vi "Advanced Cut - Auto Reverse Cut.vi"(8 "error in (no error)":errorcluster, 11 "Auto Cut (Reverse)":T1={"End Time (s)"=0.0, "# Epochs"=10, "Epoch Duration (s)"=90.0} {"Epoch Duration (s)" min=0.0 step=1.0; "End Time (s)" min=0.0 step=1.0}) -> (0 "error out":errorcluster, 3 "Snippets":dbl[][](array[numeric]))   [LabVIEW 2016]
uses:
  Type Definitions/Advanced Cut - Reverse Auto Cut.ctl
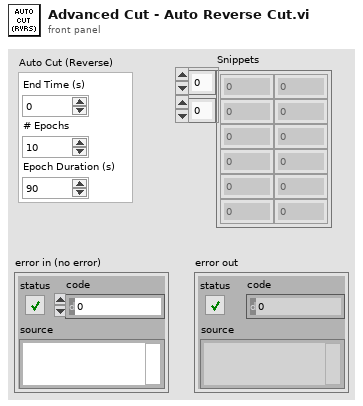
[diagram p1: front panel]
types:
  T1 = typedef "Advanced Cut - Reverse Auto Cut.ctl" = cluster{"End Time (s)":dbl, "# Epochs":u32, "Epoch Duration (s)":dbl}
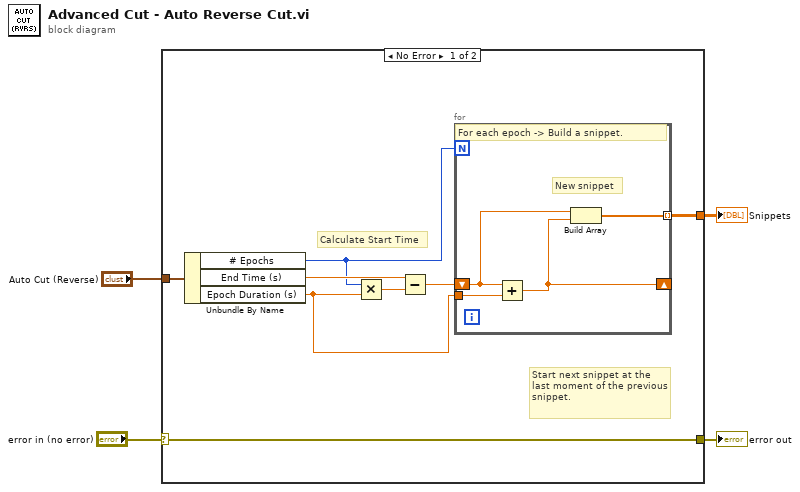
[diagram p0: block diagram]
diagram:
  n1 = case shown="No Error" "error in (no error)" {
    selector: "error in (no error)" -> [w12 w17]
    tunnel: [w12 w17] -> w3
    tunnel: [w11 _] -> w2
    tunnel: "Auto Cut (Reverse)" -> [w10 _]
    frame No Error {
      # "Calculate Start Time"
      # "Start next snippet at the last moment of the previous snippet."
      n2 = Unbundle By Name(w10) -> ("# Epochs"=w6:u32, "End Time (s)"=w9:dbl, "Epoch Duration (s)"=w7:dbl)
      n3 = Multiply(x=w6, y=w7) -> (x*y=w5:dbl)
      n4 = Subtract(x=w9, y=w5) -> (x-y=w8:dbl)
      n5 = for {
        N: w6 -> [_]
        shift-right: [w15] -> _
        shift-left: w8 -> [w16]
        tunnel: [w14] -> w11 mode=indexing
        tunnel: w7 -> [w13]
        # "New snippet"
        # "For each epoch -> Build a snippet."
        n6 = Add(x=w16, y=w13) -> (x+y=w15:dbl)
        n7 = Build Array(w16, w15) -> (w14:dbl[])
      }
    }
    frame Error {
    }
  }
  "error out" <- w3
  "Snippets" <- w2
